vi "Lab3_chirp_part2.vi"() -> ()   [LabVIEW 2010]
uses:
  <vilib>/Analysis/NI_AALBase.lvlib
  <vilib>/measure/NI_MABase.lvlib
  <vilib>/Analysis/NI_AALPro.lvlib
panel:
  in  "phase":dbl(knob) scale=0.0..90.0
  out "Modulated Chirp":waveform(dbl)(graph)
  in  "FM mod Index":dbl(slide) scale=0.0..0.01
  out "Chirp":dbl[](graph)
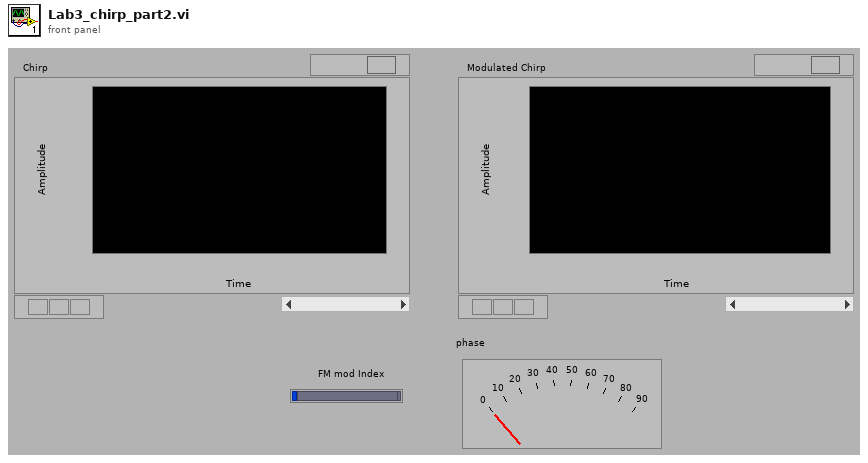
[diagram p1: front panel]
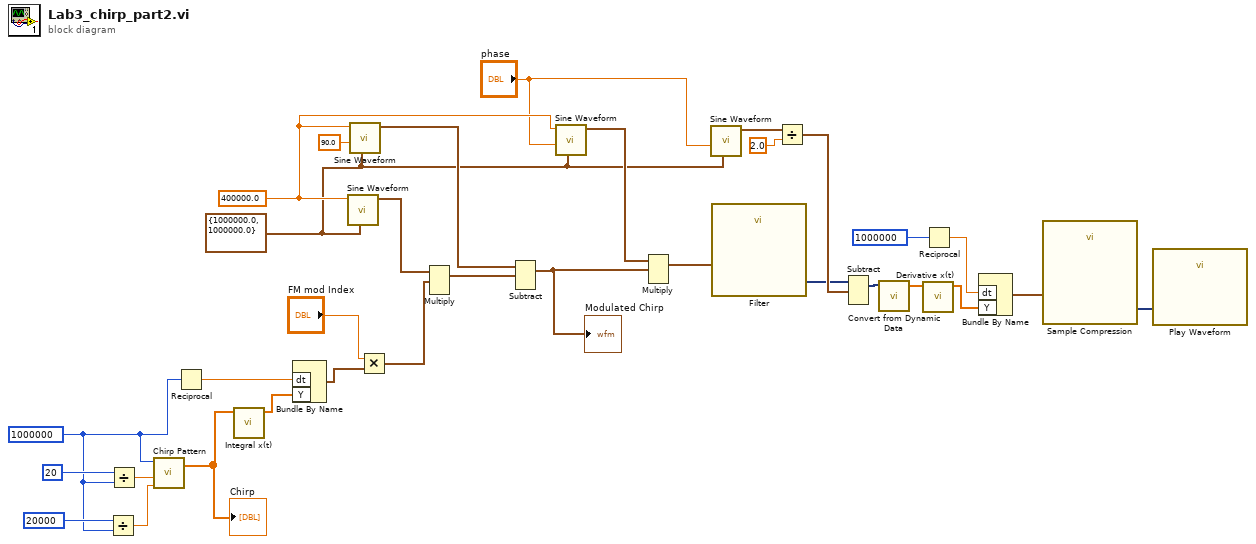
[diagram p0: block diagram]
diagram:
  w19 = cluster{"Fs":dbl, "#s":dbl} {"Fs"=1000000.0, "#s"=1000000.0} ("sampling info")
  w23 = 400000.0 ("frequency")
  w28 = 1000000 ("samples")
  n1 = Divide(x=20000 ("samples"), y=w28) -> (x/y=w30:dbl)
  n2 = Divide(x=20 ("samples"), y=w28) -> (x/y=w32:dbl)
  n3 = call <vilib>:"Chirp Pattern.vi"("f2"=w30, "f1"=w32, "samples"=w28) -> ("Chirp Pattern"=w12:dbl[])  [unwired: 1 in, 1 out]
  "Chirp" <- w12
  n4 = Reciprocal(x=w28) -> (1/x=w6:dbl)
  n5 = call <vilib>:"Integral x(t).vi"("X"=w12) -> ("Integral X"=w13:dbl[])  [unwired: 9 in, 1 out]
  n6 = Bundle By Name("dt"=w6, "Y"=w13) -> (w5:waveform(dbl))  [unwired: 1 in]
  n7 = call <vilib>:"Sine Waveform.vi"("sampling info"=w19, "frequency"=w23) -> ("signal out"=w26:waveform(dbl))  [unwired: 8 in, 1 out]
  n8 = call <vilib>:"Sine Waveform.vi"("sampling info"=w19, "phase"=90.0, "frequency"=w23) -> ("signal out"=w24:waveform(dbl))  [unwired: 7 in, 1 out]
  n9 = Multiply(x="FM mod Index", y=w5) -> (x*y=w14:waveform(dbl))
  n10 = Multiply(1:w14, 2:w26) -> (0:w25:waveform(dbl))  [unwired: 1 in, 1 out]
  n11 = Subtract(1:w25, 2:w24) -> (0:w22:waveform(dbl))  [unwired: 1 in, 1 out]
  "Modulated Chirp" <- w22
  n12 = call <vilib>:"Sine Waveform.vi"("sampling info"=w19, "phase"="phase", "frequency"=w23) -> ("signal out"=w21:waveform(dbl))  [unwired: 7 in, 1 out]
  n13 = Multiply(1:w22, 2:w21) -> (0:w20:waveform(dbl))  [unwired: 1 in, 1 out]
  n14 = call <vilib>:"Sine Waveform.vi"("sampling info"=w19, "phase"="phase") -> ("signal out"=w18:waveform(dbl))  [unwired: 8 in, 1 out]
  n15 = call "Filter"("Signal"=w20) -> ("Filtered Signal"=w4:dynamicdata)  [unwired: 9 in, 1 out]
  n16 = Divide(x=w18, y=2.0) -> (x/y=w16:waveform(dbl))
  n17 = Subtract(1:w16, 2:w4) -> (0:w11:dynamicdata)  [unwired: 1 in, 1 out]
  n18 = call "Convert from Dynamic Data"("Dynamic Data Type"=w11) -> ("Array"=w10:dbl[])  [unwired: 3 in]
  n19 = call <vilib>:"Derivative x(t).vi"("X"=w10) -> ("dX/dt"=w8:dbl[])  [unwired: 9 in, 1 out]
  n20 = Reciprocal(x=1000000 ("samples")) -> (1/x=w9:dbl)
  n21 = Bundle By Name("dt"=w9, "Y"=w8) -> (w3:waveform(dbl))  [unwired: 1 in]
  n22 = call "Sample Compression"("Signals"=w3) -> ("Mean"=w1:dynamicdata)  [unwired: 8 in, 2 out]
  n23 = call "Play Waveform"("Data"=w1) -> ()  [unwired: 18 in, 1 out]
